vi "Robot Turn (William + Michael S).vi"(7 "Reset":bool, 8 "Desired Time":dbl=4.0, 9 "X axis value":dbl=0.3, 10 "Desired Degree":dbl=180.0, 11 "Gyro Degrees":dbl=0.0600058532304) -> (3 "Stop":bool=TRUE, 6 "Rotational Value":dbl)   [LabVIEW 2015]
uses:
  Turn State.ctl
panel:
  out "Turn Right?":bool=TRUE
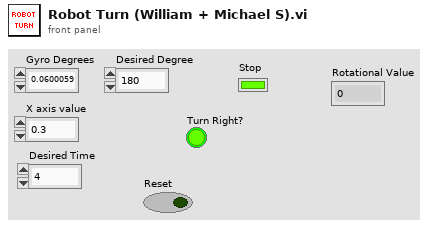
[diagram p1: front panel]
types:
  T1 = typedef "Turn State.ctl" = enum16{"Reset Encoder", "Determine Direction", "Turn Robot", "Stop"}
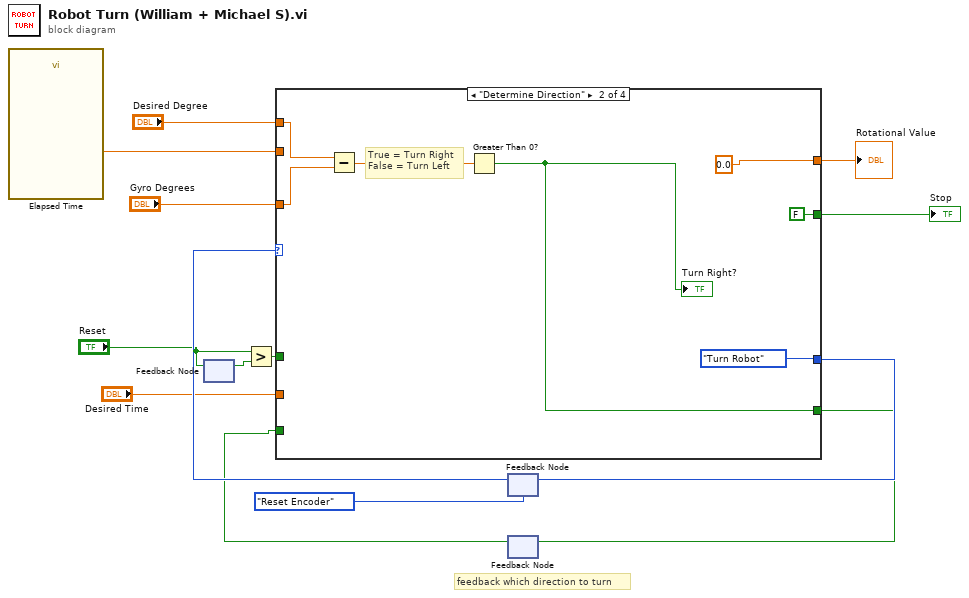
[diagram p0: block diagram]
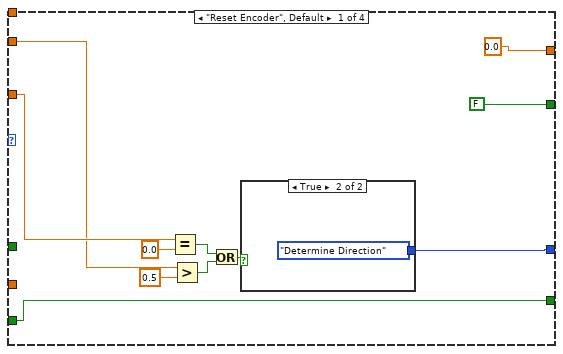
[diagram p2: hidden frame]
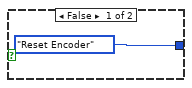
[diagram p3: hidden frame]
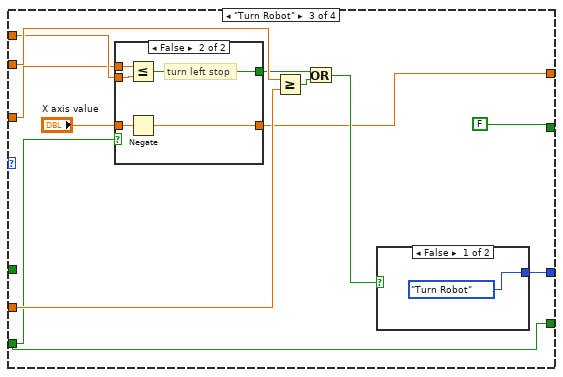
[diagram p4: hidden frame]
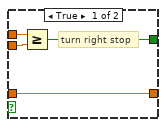
[diagram p5: hidden frame]
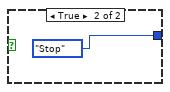
[diagram p6: hidden frame]
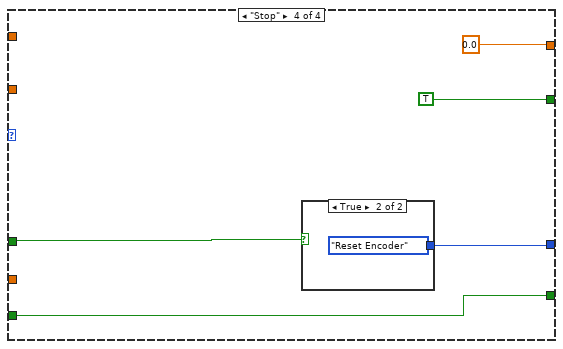
[diagram p7: hidden frame]
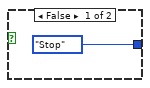
[diagram p8: hidden frame]
diagram:
  # "feedback which direction to turn"
  n1 = call "Elapsed Time"() -> ("Elapsed Time (s)"=w11:dbl)  [unwired: 12 in, 7 out]
  n2 = feedback-in #1("Reset") -> ()
  n3 = feedback #1() -> (w4:bool)  [unwired: 1 in]
  n4 = Greater?(x="Reset", y=w4) -> (0:w2:bool)
  n5 = feedback #2(Turn_State."Reset Encoder") -> (w13:T1)
  n6 = feedback #3() -> (w5:bool)  [unwired: 1 in]
  n7 = case shown="\"Determine Direction\"" w13 {
    tunnel: "Gyro Degrees" -> [w25 w33 w39 _]
    tunnel: w11 -> [w23 _ w46 _]
    tunnel: [w19 Turn_State."Turn Robot" w43 w62] -> w10
    tunnel: "Desired Degree" -> [_ w34 w40 _]
    tunnel: [FALSE FALSE FALSE TRUE] -> w8
    tunnel: "Desired Time" -> [_ _ w41 _]
    tunnel: [w16 w29 w36 w60] -> w6
    tunnel: w5 -> [w16 _ w36 w60]
    tunnel: w2 -> [_ _ _ w59]
    tunnel: [0.0 0.0 w35 0.0] -> w1
    frame "Reset Encoder", Default {
      n8 = Equal?(x=w25, y=0.0) -> (x = y?=w21:bool)
      n9 = Greater?(x=w23, y=0.5) -> (0:w22:bool)
      n10 = Or(x=w21, y=w22) -> (x .or. y?=w20:bool)
      n11 = case shown="True" w20 {
        tunnel: [Turn_State."Reset Encoder" Turn_State."Determine Direction"] -> w19
        frame False {
        }
        frame True {
        }
      }
    }
    frame "Determine Direction" {
      # "True = Turn Right\nFalse = Turn Left"
      n12 = Subtract(x=w34, y=w33) -> (x-y=w32:dbl)
      n13 = Greater Than 0?(x=w32) -> (x > 0?=w29:bool)
      "Turn Right?" <- w29
    }
    frame "Turn Robot" {
      n14 = case shown="False" w36 {
        tunnel: w40 -> [w49 w54]
        tunnel: w39 -> [w50 w55]
        tunnel: [w48 w53] -> w38
        tunnel: "X axis value" -> [w47 w52]
        tunnel: [w47 w51] -> w35
        frame True {
          # "turn right stop"
          n15 = Greater Or Equal?(x=w50, y=w49) -> (x >= y?=w48:bool)
        }
        frame False {
          # "turn left stop"
          n16 = Less Or Equal?(x=w55, y=w54) -> (x <= y?=w53:bool)
          n17 = Negate(x=w52) -> (-x=w51:dbl)
        }
      }
      n18 = Greater Or Equal?(x=w46, y=w41) -> (x >= y?=w45:bool)
      n19 = Or(x=w38, y=w45) -> (x .or. y?=w44:bool)
      n20 = case shown="False" w44 {
        tunnel: [Turn_State."Turn Robot" Turn_State."Stop"] -> w43
        frame False {
        }
        frame True {
        }
      }
    }
    frame "Stop" {
      n21 = case shown="True" w59 {
        tunnel: [Turn_State."Stop" Turn_State."Reset Encoder"] -> w62
        frame False {
        }
        frame True {
        }
      }
    }
  }
  "Stop" <- w8
  "Rotational Value" <- w1
  n22 = feedback-in #2(w10) -> ()
  n23 = feedback-in #3(w6) -> ()
